vi "HFRR ADV v06.vi"() -> ()   [LabVIEW 2025] (continued)
            n2697 = Number To Fractional String(number=w3830, width (-)=i16 6, precision (6)=i16 2) -> (F-format string=w3835:string)  [unwired: 1 in]
            n2698 = Number To Fractional String(number=w3819, width (-)=i16 6, precision (6)=i16 2) -> (F-format string=w3821:string)  [unwired: 1 in]
            n2699 = Number To Fractional String(number=w3805, width (-)=i16 6, precision (6)=i16 2) -> (F-format string=w3806:string)  [unwired: 1 in]
            n2700 = Number To Fractional String(number=w3818, width (-)=i16 6, precision (6)=i16 2) -> (F-format string=w3820:string)  [unwired: 1 in]
            n2701 = Number To Fractional String(number=w3801, width (-)=i16 6, precision (6)=i16 2) -> (F-format string=w3800:string)  [unwired: 1 in]
            n2702 = Number To Fractional String(number=w3797, precision (6)=i16 2) -> (F-format string=w3796:string)  [unwired: 2 in]
            n2703 = call-dynamic "Set Report Header Text.vi"("report in"=w3839, "center header text"=w3791, "error in (no error)"=w3838) -> ("report out"=w3810:refnum<class "NI_report.lvclass">, "error out"=w3811:errorcluster)  [unwired: 11 in]
            n2704 = Concatenate Strings(w3799, w3783, w3835, w3799, w3780, w3804, w3799, w3778, w3817, w3799, w3775, w3806, w3799, w3771, w3821, w3799, w3768, w3820, w3799, w3766, w3800, w3799, w3763, w3796) -> (w3787:string)
            "export 2" <- w3787
            n2705 = call-poly <vilib>:"Append Report Text.vi"("report in"=w3810, "text"=w3809, "error in (no error)"=w3811) -> ("report out"=w3813:refnum<class "NI_report.lvclass">, "error out"=w3812:errorcluster)  [unwired: 9 in, 2 out]
            n2706 = local read "test by"() -> (w3786:string)
            n2707 = local read "TITTLE"() -> (w3788:string)
            n2708 = call-poly <vilib>:"Append Report Text.vi"("report in"=w3813, "error in (no error)"=w3812) -> ("report out"=w3834:refnum<class "NI_report.lvclass">, "error out"=w3832:errorcluster)  [unwired: 10 in, 2 out]
            n2709 = Concatenate Strings(w3788, w3787, w3786) -> (→"output":string)
            n2710 = call-poly <vilib>:"Append Report Text.vi"("report in"=w3834, "text"=w3787, "error in (no error)"=w3832) -> ("report out"=w3833:refnum<class "NI_report.lvclass">, "error out"=w3831:errorcluster)  [unwired: 9 in, 2 out]
            n2711 = call-dynamic "Print Report.vi"("report in"=w3833, "printer name (default)"=w3841, "error in (no error)"=w3831) -> ("report out"=w3843:refnum<class "NI_report.lvclass">, "error out"=w3844:errorcluster)  [unwired: 11 in]
            n2712 = call-dynamic "Dispose Report.vi"("report in"=w3843, "error in (no error)"=w3844) -> ()  [unwired: 13 in, 1 out]
          }
        }
        n2713 = case shown="True" "Print 2" {
          frame False {
          }
          frame True {
            n2714 = flat-sequence {
              frame #0 {
                n2715 = local read "s.NO"() -> (→"s.NO 2":string)
                n2716 = Wait (ms)(milliseconds to wait=u32 20) -> ()  [unwired: 1 out]
                n2717 = local read "Sample ID  3"() -> (→"Sample ID  6":string)
                n2718 = local read "Sample ID  4"() -> (→"Sample ID  7":string)
                n2719 = local read "Sample ID"() -> (→"Sample ID  2":string)
                n2720 = local read "Tested by"() -> (→"Tested by 2":string)
                n2721 = local read "Test Date"() -> (→"Test Date 2":string)
                n2722 = local read "Humidity after test 3"() -> (→"Humidity after test 4":dbl)
                n2723 = local read "Ref A Test Date :"() -> (→"TITTLE 4":string)
                n2724 = local read "Temperature before test 3"() -> (w3666:dbl)
                n2725 = local read "Temperature before test 3"() -> (→"Temperature after test 5":dbl)
                n2726 = local read "Temperature after test 3"() -> (→"Temperature after test 4":dbl)
                n2727 = local read "Humidity before test 3"() -> (→"Humidity before test 4":dbl)
                n2728 = local write "Temperature before test 3"(w3666) -> ()
                n2729 = local read "image data"() -> (w3657:T11)
                n2730 = String To Path(string="C:\\LAB-IQ\\im\\Temp_resized.jpg") -> (path=w3658:path)
                "path 2" <- w3658
                n2731 = call <vilib>:"Write JPEG File.vi"("image data"=w3657, "path to JPEG file"=w3658) -> ()  [unwired: 8 in, 2 out]
                "Ref A Test Date :" <- "Ref A Test Date :"
                "Ref B Test Date :" <- "Ref B Test Date :"
                "Ref B Scar Value :" <- "Ref B Scar Value :"
                "Ref A Scar Value :" <- "Ref A Scar Value :"
              }
              frame #1 {
                (unwired) HTML_Report_Image_Alignment."MIDDLE" ("alignment (default)")
                w3694 = u16 0 items=["portrait", "landscape"] ("orientation (portrait)")
                (unwired) HTML_Report_Image_Alignment."ABSMIDDLE" ("alignment (default)")
                (unwired) "TESTED BY : "
                (unwired) "TESTED DATE :"
                (unwired) "SAMPLE ID : "
                (unwired) "SAMPLE DESIGN : "
                w3727 = "\r"
                # "add image"
                n2732 = Wait (ms)(milliseconds to wait=u32 20) -> ()  [unwired: 1 out]
                n2733 = local read "Sample ID  2"() -> (w3720:string)
                n2734 = local read "Wear Scar X"() -> (w3692:dbl)
                "Length ( microns ) 2" <- w3692
                n2735 = local read "Wear Scar Y"() -> (w3691:dbl)
                "Wear Scar Y ( microns ) :" <- w3691
                n2736 = local read "Test Date 2"() -> (w3721:string)
                n2737 = local read "Tested by 2"() -> (w3722:string)
                n2738 = local read "String 46"() -> (w3718:string)
                n2739 = local read "String 48"() -> (w3724:string)
                n2740 = local read "String 47"() -> (w3723:string)
                n2741 = local read "String 49"() -> (w3725:string)
                n2742 = local read "String 10"() -> (w3678:string)
                n2743 = local read "s.NO 2"() -> (w3719:string)
                n2744 = Add(x=w3692, y=w3691) -> (x+y=w3690:dbl)
                n2745 = call <vilib>:"New Report.vi"("report type"=enum16{"Standard Report", "HTML"}."HTML") -> ("report out"=w3698:refnum<class "NI_report.lvclass">, "error out"=w3696:errorcluster)  [unwired: 13 in]
                n2746 = Concatenate Strings(w3727, w3718, w3719, w3727, w3724, w3720, w3727, w3723, w3721, w3727, w3725, w3722, w3727) -> (→"test by 2":string)
                n2747 = Concatenate Strings("C:\\LAB-IQ\\Data\\" ("string"), w3678, ".jpg" ("string")) -> ()  [unwired: 1 out]
                n2748 = Divide(x=w3690, y=2.0) -> (x/y=→"Mean Wear ( microns) :":dbl)
                n2749 = call-dynamic "Set Report Orientation.vi"("report in"=w3698, "orientation (portrait)"=w3694, "error in (no error)"=w3696) -> ("report out"=w3697:refnum<class "NI_report.lvclass">, "error out"=w3695:errorcluster)  [unwired: 11 in]
                n2750 = for {
                  N: 5 -> [_]
                  tunnel: w3697 -> [w3748]
                  tunnel: [w3747] -> w3676
                  tunnel: w3695 -> [w3746]
                  tunnel: [w3745] -> w3675
                  n2751 = call-dynamic "Set Report Tab Width.vi"("report in"=w3748, "error in (no error)"=w3746) -> ("report out"=w3747:refnum<class "NI_report.lvclass">, "error out"=w3745:errorcluster)  [unwired: 12 in]
                }
                n2752 = local read "TITTLE"() -> (w3693:string)
                n2753 = call-dynamic "Set Report Header Text.vi"("report in"=w3676, "center header text"=w3693, "error in (no error)"=w3675) -> ("report out"=w3714:refnum<class "NI_report.lvclass">, "error out"=w3713:errorcluster)  [unwired: 11 in]
                n2754 = for {
                  N: 1 -> [_]
                  tunnel: [w3752] -> w3700
                  tunnel: [w3751] -> w3699
                  tunnel: w3714 -> [w3750]
                  tunnel: w3713 -> [w3749]
                  n2755 = call-dynamic "New Report Line.vi"("report in"=w3750, "error in (no error)"=w3749) -> ("report out"=w3752:refnum<class "NI_report.lvclass">, "error out"=w3751:errorcluster)  [unwired: 12 in]
                }
                n2756 = for {
                  N: 2 -> [_]
                  tunnel: [w3744] -> w3706
                  tunnel: [w3743] -> w3705
                  tunnel: w3700 -> [w3742]
                  tunnel: w3699 -> [w3741]
                  n2757 = call-dynamic "New Report Line.vi"("report in"=w3742, "error in (no error)"=w3741) -> ("report out"=w3744:refnum<class "NI_report.lvclass">, "error out"=w3743:errorcluster)  [unwired: 12 in]
                }
                n2758 = for {
                  N: 25 -> [_]
                  tunnel: w3706 -> [w3740]
                  tunnel: w3705 -> [w3738]
                  tunnel: [w3739] -> w3709
                  tunnel: [w3737] -> w3708
                  n2759 = call-dynamic "Set Report Tab Width.vi"("report in"=w3740, "error in (no error)"=w3738) -> ("report out"=w3739:refnum<class "NI_report.lvclass">, "error out"=w3737:errorcluster)  [unwired: 12 in]
                }
                n2760 = control-ref of="Tab Control 9"() -> (w3704:refnum<vi>)
                n2761 = call-dynamic "Append Control Image to Report.vi"("report in"=w3709, "alignment (default)"=HTML_Report_Image_Alignment."ABSMIDDLE", "ctrl reference"=w3704, "error in (no error)"=w3708) -> ("report out"=w3703:refnum<class "NI_report.lvclass">, "error out"=w3702:errorcluster)  [unwired: 8 in, 2 out]
                n2762 = for {
                  N: 3 -> [_]
                  tunnel: [w3736] -> w3687
                  tunnel: [w3735] -> w3686
                  tunnel: w3703 -> [w3734]
                  tunnel: w3702 -> [w3733]
                  n2763 = call-dynamic "New Report Line.vi"("report in"=w3734, "error in (no error)"=w3733) -> ("report out"=w3736:refnum<class "NI_report.lvclass">, "error out"=w3735:errorcluster)  [unwired: 12 in]
                }
                n2764 = for {
                  N: 100 -> [_]
                  tunnel: w3687 -> [w3732]
                  tunnel: w3686 -> [w3730]
                  tunnel: [w3731] -> w3683
                  tunnel: [w3729] -> w3681
                  n2765 = call-dynamic "Set Report Tab Width.vi"("report in"=w3732, "error in (no error)"=w3730) -> ("report out"=w3731:refnum<class "NI_report.lvclass">, "error out"=w3729:errorcluster)  [unwired: 12 in]
                }
                n2766 = String To Path(string="C:\\LAB-IQ\\im\\Temp_resized.jpg") -> (path=w3673:path)
                n2767 = call-poly <vilib>:"Append Image to Report.vi"("report in"=w3683, "path or URL of image"=w3673, "error in (no error)"=w3681) -> ("report out"=w3682:refnum<class "NI_report.lvclass">, "error out"=w3680:errorcluster)  [unwired: 9 in, 2 out]
                n2768 = call-poly <vilib>:"Open HTML Report in Browser.vi"("report in"=w3682, "error in (no error)"=w3680) -> ("report out"=w3717:refnum<class "NI_report.lvclass">, "error out"=w3716:errorcluster)  [unwired: 11 in, 1 out]
                n2769 = call-dynamic "Dispose Report.vi"("report in"=w3717, "error in (no error)"=w3716) -> ()  [unwired: 13 in, 1 out]
              }
              frame #2 {
              }
              frame #3 {
                n2770 = disable-structure shown="Disabled" {
                  frame Disabled {
                    n2771 = local read "String 10"() -> (w3757:string)
                    n2772 = Concatenate Strings("C:\\LAB-IQ-NXT\\Data\\" ("string"), w3757, ".jpg" ("string")) -> (w3755:string)
                    n2773 = String To Path(string=w3755) -> (path=w3754:path)
                    n2774 = Delete(path (use dialog)=w3754) -> ()  [unwired: 4 in, 3 out]
                  }
                  frame Enabled {
                  }
                }
                n2775 = local write "Print 2"(FALSE ("Print")) -> ()
              }
            }
          }
        }
      }
    }
    n2776 = property on="SetTemp" class="DigNum (strict)"("Disabled"=w1732) -> ()  [unwired: 2 in, 2 out]
    n2777 = Multiply(x=w1721, y=w1723) -> (x*y=w1722:dbl)
    n2778 = local read "MWSD"() -> (w1720:dbl)
    n2779 = Add(x=w1722, y=w1720) -> (x+y=→"WS1.4":dbl)
    n2780 = Wait (ms)(milliseconds to wait=u32 50) -> ()  [unwired: 1 out]
    n2781 = Wait (ms)(milliseconds to wait=u32 50) -> ()  [unwired: 1 out]
    n2782 = local read "Quit"() -> (w1719:bool)
  }
  n2783 = VISA Close(VISA resource name=w44, error in (no error)=w43) -> (error out=w41:errorcluster)
  n2784 = VISA Close(VISA resource name=w25, error in (no error)=w24) -> ()  [unwired: 1 out]
  n2785 = call <vilib>:"Clear Errors.vi"("error in (no error)"=w41) -> ()  [unwired: 5 in, 2 out]
  n2786 = Or(x=w31, y=w30) -> (x .or. y?=w32:bool)
  n2787 = while {
    tunnel: [w3905] -> w37
    shift-right: [w3943] -> _
    shift-left: "" -> [w3931]
    tunnel: [w3919] -> _
    i -> [w3919]
    stop <- w3905 stop-if-true
    w3945 = ";" ("string")
    n2788 = local read "start en"() -> (w3964:bool)
    n2789 = And(x="st enable", y=w3964) -> (x .and. y?=w3965:bool)
    n2790 = local read "ACQUIRE 3"() -> (w3908:bool)
    n2791 = local read "Elapsed time"() -> (w3927:dbl)
    n2792 = case shown="True" w3965 {
      tunnel: "st enable" -> [w4029 w4030]
      tunnel: [w4029 w4030] -> w3909
      frame False {
      }
      frame True {
        n2793 = local write "start en"(FALSE ("start en")) -> ()
      }
    }
    n2794 = Wait (ms)(milliseconds to wait=u32 80) -> ()  [unwired: 1 out]
    n2795 = local read "Stroke"() -> (w3918:dbl)
    n2796 = Greater?(x=w3927, y=0.1) -> (0:w3925:bool)
    n2797 = Or(x=w3909, y=w3908) -> (x .or. y?=w3910:bool)
    n2798 = case shown="True" "ACQUIRE 2" {
      frame False {
      }
      frame True {
        n2799 = call "Elapsed Time13"() -> ("Time has Elapsed"=w3972:bool)  [unwired: 12 in, 7 out]
        n2800 = case shown="True" w3972 {
          frame False {
          }
          frame True {
            n2801 = local write "ACQUIRE 2"(FALSE ("ACQUIRE 2")) -> ()
            n2802 = local write "ACQUIRE 3"(FALSE ("ACQUIRE 2")) -> ()
          }
        }
        n2803 = local write "ACQUIRE 3"(TRUE ("ACQUIRE 2")) -> ()
      }
    }
    n2804 = case shown="True" w3910 {
      tunnel: w3918 -> [_ w4052]
      tunnel: [w4032 _] -> w3962
      tunnel: w3925 -> [_ _]
      tunnel: w3908 -> [_ w4039]
      frame False {
        w4032 = TRUE ("PID Rst")
        n2805 = local read "stop cmd"() -> (w4033:bool)
        n2806 = case shown="True" w4033 {
          frame False {
          }
          frame True {
            n2807 = local write "stop cmd"(FALSE ("stop cmd")) -> ()
          }
        }
        n2808 = local write "PID Rst"(TRUE ("PID Rst")) -> ()
        "start en" <- w4032
      }
      frame True {
        w4059 = cluster{"output high":dbl, "output low":dbl} {"output high"=600.0, "output low"=-600.0} ("output range")
        n2809 = local read "STROKE GAIN :"() -> (w4044:dbl)
        n2810 = call "Elapsed Time6"("Reset"="PID Rst", "Auto Reset"=FALSE) -> ("Time has Elapsed"=w4053:bool)  [unwired: 10 in, 7 out]
        n2811 = Multiply(x="Set Strk", y=w4044) -> (x*y=w4037:dbl)
        n2812 = case shown="False" w4053 {
          tunnel: [w4064 w4065] -> w4056
          tunnel: "Set Strk" -> [w4064 _]
          tunnel: w4052 -> [_ w4065]
          frame False {
          }
          frame True {
          }
        }
        n2813 = Multiply(x=w4037, y=1.0) -> (x*y=w4036:dbl)
        n2814 = Select(t=T8 {"Proportional Gain (Kc)"=0.0, "Integral Time (Ti, min)"=0.02, "Derivative Time (Td, min)"=0.0} ("Stroke PID Gains"), s=w4039, f="Stroke PID Gains") -> (s? t:f=w4040:T8)
        n2815 = Not(x=w4053) -> (.not. x?=w4051:bool)
        n2816 = call-poly <vilib>:"PID.vi"("reinitialize? (F)"=w4051, "output range"=w4059, "PID gains"=w4040, "process variable"=w4056, "setpoint"="Set Strk") -> ("output"=w4050:dbl)  [unwired: 5 in, 1 out]
        "Slide 5" <- w4050
        n2817 = Select(t=w4050, s=w4053, f=0.0) -> (s? t:f=w4054:dbl)
        n2818 = flat-sequence {
          tunnel: w4054 -> [_]
          frame #0 {
            n2819 = local write "PID Rst"(FALSE ("PID Rst")) -> ()
          }
        }
        n2820 = Add(x=w4036, y=w4054) -> (x+y=w4049:dbl)
        n2821 = Unbundle(w4059) -> ("output high"=w4058:dbl, "output low"=w4057:dbl)
        n2822 = To Word Integer(number=w4049) -> (16bit integer=w4046:i16)
        n2823 = property on="Slide 5" class="Slide (strict)"("Scale.Range:Minimum"=w4057, "Scale.Range:Maximum"=w4058) -> ()  [unwired: 2 in, 2 out]
        n2824 = In Range and Coerce(upper limit=4095.0 ("f"), x=w4046, lower limit=100.0 ("f")) -> (coerced(x)=w4043:dbl)  [unwired: 1 out]
        "PID Out" <- w4043
        n2825 = Number To Decimal String(number=w4043) -> (decimal integer string=→"st gain":string)  [unwired: 1 in]
        "stop cmd" <- TRUE ("Auto Reset")
      }
    }
    n2826 = flat-sequence {
      frame #0 {
        n2827 = local read "CH-POWER +"() -> (w3976:u16)
        n2828 = local read "CH-POWER -"() -> (w3977:u16)
        n2829 = case shown="1" w3977 {
          tunnel: "PWR" -> [w3978 w3979 w3980 w3981 w3982 w3983 w3984 w3985]
          frame 0, Default {
            n2830 = local write "Do 0"(w3978) -> ()
          }
          frame 1 {
            n2831 = local write "Do 1"(w3979) -> ()
          }
          frame 2 {
            n2832 = local write "Do 2"(w3980) -> ()
          }
          frame 3 {
            n2833 = local write "Do 3"(w3981) -> ()
          }
          frame 4 {
            n2834 = local write "Do 4"(w3982) -> ()
          }
          frame 5 {
            n2835 = local write "Do 5"(w3983) -> ()
          }
          frame 6 {
            n2836 = local write "Do 6"(w3984) -> ()
          }
          frame 7 {
            n2837 = local write "Do 7"(w3985) -> ()
          }
        }
        n2838 = case shown="1" w3976 {
          tunnel: "PWR" -> [w3986 w3987 w3988 w3989 w3990 w3991 w3992 w3993]
          frame 0, Default {
            n2839 = local write "Do 0"(w3986) -> ()
          }
          frame 1 {
            n2840 = local write "Do 1"(w3987) -> ()
          }
          frame 2 {
            n2841 = local write "Do 2"(w3988) -> ()
          }
          frame 3 {
            n2842 = local write "Do 3"(w3989) -> ()
          }
          frame 4 {
            n2843 = local write "Do 4"(w3990) -> ()
          }
          frame 5 {
            n2844 = local write "Do 5"(w3991) -> ()
          }
          frame 6 {
            n2845 = local write "Do 6"(w3992) -> ()
          }
          frame 7 {
            n2846 = local write "Do 7"(w3993) -> ()
          }
        }
      }
    }
    n2847 = local read "RUN"() -> (w3916:bool)
    n2848 = Or(x=w3916, y="ACQUIRE 3") -> (x .or. y?=w3915:bool)
    n2849 = local read "Set Hz"() -> (w3933:dbl)
    n2850 = Select(t=w3933, s=w3915, f=0.0) -> (s? t:f=w3932:dbl)
    n2851 = local read "st gain"() -> (w3936:string)
    n2852 = local read "DO"() -> (w3937:string)
    n2853 = case shown="True" "Boolean 10" {
      frame False {
      }
      frame True {
        n2854 = local write "Tab Control 8"(enum32{"setup", "calibrate"}."calibrate" ("Tab Control 8")) -> ()
        n2855 = local write "Boolean 10"(FALSE ("Boolean 10")) -> ()
      }
    }
    n2856 = Number To Decimal String(number=w3932) -> (decimal integer string=w3935:string)  [unwired: 1 in]
    n2857 = case shown="True" "Boolean 11" {
      frame False {
      }
      frame True {
        n2858 = local write "Tab Control 8"(enum32{"setup", "calibrate"}."setup" ("Tab Control 8")) -> ()
        n2859 = local write "Boolean 11"(FALSE ("Boolean 11")) -> ()
      }
    }
    n2860 = String Length(string=w3936) -> (length=w3951:i32)
    n2861 = String Length(string=w3937) -> (length=w3939:i32)
    n2862 = String Length(string=w3935) -> (length=w3952:i32)
    n2863 = Subtract(x=4.0, y=w3951) -> (x-y=w3948:dbl)
    n2864 = Subtract(x=3.0, y=w3939) -> (x-y=w3942:dbl)
    n2865 = flat-sequence {
      tunnel: w3962 -> [_]
      frame #0 {
        n2866 = Build Array("Do 0", "Do 1", "Do 2", "Do 3", "Do 4", "Do 5", "Do 6", "Do 7") -> (w4020:bool[])
        n2867 = Boolean Array To Number(Boolean array=w4020) -> (number=w4018:u32)
        n2868 = Add(x=w4018, y=u32 0) -> (x+y=w4016:u32)
        n2869 = Number To Decimal String(number=w4016) -> (decimal integer string=→"DO":string)  [unwired: 1 in]
      }
    }
    n2870 = Subtract(x=3.0, y=w3952) -> (x-y=w3953:dbl)
    n2871 = Replace Substring(3:w3948, 4:w3936, 5:"0000" ("string")) -> (1:w3946:string)  [unwired: 1 in, 1 out]
    n2872 = Replace Substring(3:w3942, 4:w3937, 5:"000" ("string")) -> (1:w3938:string)  [unwired: 1 in, 1 out]
    n2873 = Replace Substring(3:w3953, 4:w3935, 5:"000" ("string")) -> (1:w3947:string)  [unwired: 1 in, 1 out]
    n2874 = Concatenate Strings("*" ("string"), w3947, w3945, w3946, w3945, w3938, "$" ("string")) -> (w3943:string)
    "Stroke_send_Val" <- w3943
    n2875 = local read "RUN"() -> (w3913:bool)
    n2876 = local read "ACQUIRE 3"() -> (w3912:bool)
    n2877 = local read "send"() -> (w3929:bool)
    n2878 = Not Equal?(x=w3931, y=w3943) -> (x != y?=w3944:bool)
    n2879 = Or(x=w3913, y=w3912) -> (x .or. y?=w3911:bool)
    n2880 = And(x=w3929, y=w3911) -> (x .and. y?=w3928:bool)
    n2881 = Or(x=w3944, y=w3928) -> (x .or. y?=w3922:bool)
    n2882 = case shown="False" w3911 {
      frame False {
        "send" <- TRUE ("send")
      }
      frame True {
      }
    }
    n2883 = call "Elapsed Time4"("Time Target (s)"=0.5) -> ("Time has Elapsed"=w3920:bool)  [unwired: 11 in, 7 out]
    n2884 = local read "Din"() -> (w3961:u8[])
    n2885 = Or(x=w3920, y=w3922) -> (x .or. y?=w3921:bool)
    n2886 = local read "Quit"() -> (w3905:bool)
    n2887 = Index Array(array=w3961, index=0) -> (element=w3959:u8)
    n2888 = case shown="True" w3921 {
      tunnel: w3943 -> [_ w3997]
      frame False {
      }
      frame True {
        n2889 = local read "Due Com"() -> (w3998:string[])
        n2890 = Build Array (concatenate)(w3998, w3997) -> (→"Due Com":string[])
        n2891 = local write "send"(FALSE ("send")) -> ()
      }
    }
    n2892 = Number To Boolean Array(number=w3959) -> (Boolean array=w3958:bool[])
    n2893 = Array Size(array=w3958) -> (size(s)=w3957:i32)
    n2894 = Greater Than 0?(x=w3957) -> (x > 0?=w3956:bool)
    n2895 = case shown="True" w3956 {
      tunnel: w3958 -> [_ w4012]
      frame False {
      }
      frame True {
        n2896 = Index Array(array=w4012, index #1=0 ("index"), index #2=1 ("index"), index #3=2 ("index"), index #4=3 ("index"), index #5=4 ("index"), index #6=5 ("index"), index #7=6 ("index"), index #8=7 ("index")) -> (element #1=→"DI 0":bool, element #2=→"DI 1":bool, element #3=→"DI 2":bool, element #4=→"DI 3":bool, element #5=→"DI 4":bool, element #6=→"DI 5":bool, element #7=→"DI 6":bool, element #8=→"DI 7":bool)
      }
    }
  }
  n2897 = Or(x=w27, y=w32) -> (x .or. y?=w39:bool)
  n2898 = control-ref of="new picture"() -> ()  [unwired: 1 out]
  n2899 = Or(x=w46, y=w39) -> (x .or. y?=w36:bool)
  n2900 = Or(x=w36, y=w37) -> (x .or. y?=w28:bool)
  n2901 = while {
    tunnel: [w4067] -> w50
    tunnel: [w4068] -> _
    i -> [w4068]
    stop <- w4067 stop-if-true
    n2902 = local read "PID-out"() -> (w4069:dbl)
    "Horizontal Slider Control" <- w4069
    n2903 = Greater Or Equal?(x=w4069, y=2.0) -> (x >= y?=w4070:bool)
    n2904 = flat-sequence {
      tunnel: w4070 -> [w4078]
      tunnel: w4069 -> [w4081]
      tunnel: [w4079] -> w4076
      tunnel: [w4077] -> w4075
      tunnel: [w4097] -> w4074
      tunnel: w4076 -> [w4097]
      tunnel: w4075 -> [w4094]
      tunnel: [w4094] -> w4073
      tunnel: w4074 -> [w4099]
      tunnel: [w4098] -> w4072
      tunnel: w4073 -> [w4098]
      tunnel: w4072 -> [w4113]
      frame #0 {
        n2905 = case shown="True" w4078 {
          selector: w4078 -> [w4083 _]
          frame False {
            n2906 = local write "HEATER"(w4083) -> ()
          }
          frame True {
            w4085 = TRUE ("data")
            n2907 = local read "CH-HEATER"() -> (w4084:u16)
            n2908 = case shown="2" w4084 {
              tunnel: w4085 -> [w4086 w4087 w4088 w4089 w4090 w4091 w4092 w4093]
              frame 0, Default {
                n2909 = local write "Do 0"(w4086) -> ()
              }
              frame 1 {
                n2910 = local write "Do 1"(w4087) -> ()
              }
              frame 2 {
                n2911 = local write "Do 2"(w4088) -> ()
              }
              frame 3 {
                n2912 = local write "Do 3"(w4089) -> ()
              }
              frame 4 {
                n2913 = local write "Do 4"(w4090) -> ()
              }
              frame 5 {
                n2914 = local write "Do 5"(w4091) -> ()
              }
              frame 6 {
                n2915 = local write "Do 6"(w4092) -> ()
              }
              frame 7 {
                n2916 = local write "Do 7"(w4093) -> ()
              }
            }
            "HEATER" <- w4085
          }
        }
        n2917 = Select(t=w4081, s=w4078, f=0.0) -> (s? t:f=w4077:dbl)
        n2918 = Greater Or Equal?(x=w4081, y=97.0) -> (x >= y?=w4079:bool)
      }
      frame #1 {
        n2919 = Multiply(x=w4094, y=5.0) -> (x*y=w4096:dbl)
        n2920 = Wait (ms)(milliseconds to wait=w4096) -> ()  [unwired: 1 out]
      }
      frame #2 {
        n2921 = case shown="False" w4099 {
          frame False {
            w4100 = FALSE ("data")
            n2922 = local read "CH-HEATER"() -> (w4101:u16)
            n2923 = case shown="4" w4101 {
              tunnel: w4100 -> [w4102 w4103 w4104 w4105 w4106 w4107 w4108 w4109]
              frame 0, Default {
                n2924 = local write "Do 0"(w4102) -> ()
              }
              frame 1 {
                n2925 = local write "Do 1"(w4103) -> ()
              }
              frame 2 {
                n2926 = local write "Do 2"(w4104) -> ()
              }
              frame 3 {
                n2927 = local write "Do 3"(w4105) -> ()
              }
              frame 4 {
                n2928 = local write "Do 4"(w4106) -> ()
              }
              frame 5 {
                n2929 = local write "Do 5"(w4107) -> ()
              }
              frame 6 {
                n2930 = local write "Do 6"(w4108) -> ()
              }
              frame 7 {
                n2931 = local write "Do 7"(w4109) -> ()
              }
            }
            n2932 = local write "HEATER"(w4100) -> ()
          }
          frame True {
          }
        }
      }
      frame #3 {
        n2933 = Subtract(x=100, y=w4113) -> (x-y=w4112:dbl)
        n2934 = Multiply(x=w4112, y=5.0) -> (x*y=w4110:dbl)
        n2935 = Wait (ms)(milliseconds to wait=w4110) -> ()  [unwired: 1 out]
      }
    }
    n2936 = local read "Quit"() -> (w4067:bool)
  }
  n2937 = Or(x=w50, y=w28) -> (x .or. y?=w49:bool)
  n2938 = while {
    tunnel: [w4115] -> w45
    i -> [w4122]
    stop <- w4115 stop-if-true
    n2939 = local read "Quit"() -> (w4115:bool)
    n2940 = Equal To 0?(x=w4122) -> (x = 0?=w4120:bool)
    n2941 = call "Elapsed Time3"("Time Target (s)"=45.0, "Auto Reset"=TRUE) -> ("Time has Elapsed"=w4119:bool)  [unwired: 10 in, 7 out]
    n2942 = Wait (ms)(milliseconds to wait=u32 50) -> ()  [unwired: 1 out]
    n2943 = Or(x=w4119, y=w4120) -> (x .or. y?=w4121:bool)
    n2944 = case shown="True" w4121 {
      frame False {
      }
      frame True {
        n2945 = call <vilib>:"System Exec.vi"("run minimized? (F)"=TRUE, "error in (no error)"="error in (no error)", "command line"="powercfg.exe -change -monitor-timeout-ac 0") -> ("error out"=w4133:errorcluster)  [unwired: 5 in, 3 out]
        n2946 = call <vilib>:"System Exec.vi"("run minimized? (F)"=TRUE, "error in (no error)"=w4133, "command line"="powercfg.exe -change -disk-timeout-ac 0") -> ("error out"=w4132:errorcluster)  [unwired: 5 in, 3 out]
        n2947 = call <vilib>:"System Exec.vi"("run minimized? (F)"=TRUE, "error in (no error)"=w4132, "command line"="powercfg.exe -change -standby-timeout-ac 0") -> ("error out"=w4131:errorcluster)  [unwired: 5 in, 3 out]
        n2948 = call <vilib>:"System Exec.vi"("run minimized? (F)"=TRUE, "error in (no error)"=w4131, "command line"="powercfg.exe -change -hibernate-timeout-ac 0") -> ("error out"=w4130:errorcluster)  [unwired: 5 in, 3 out]
        n2949 = call <vilib>:"Simple Error Handler.vi"("error in (no error)"=w4130) -> ("error out"=w4136:errorcluster)  [unwired: 4 in, 4 out]
        n2950 = call <vilib>:"Clear Errors.vi"("error in (no error)"=w4136) -> ("error out"=→"error out":errorcluster)  [unwired: 5 in, 1 out]
      }
    }
  }
  n2951 = Compound Arithmetic op=OR(w48, w49, w45) -> (w47:bool)
  n2952 = flat-sequence {
    tunnel: w47 -> [_]
    tunnel: [w4138] -> w3
    tunnel: w3 -> [_]
    frame #0 {
      n2953 = call "CLOSE CONNECTION.vi"() -> ("error out"=w4138:errorcluster)  [unwired: 11 in]
    }
    frame #1 {
      n2954 = Quit LabVIEW(quit? (T)=TRUE) -> ()
      n2955 = local write "Quit"(FALSE ("EXIT")) -> ()
    }
  }
  n2956 = property on="Heater Button" class="Bool (strict)"("Visible"=TRUE) -> ()  [unwired: 2 in, 2 out]
  n2957 = disable-structure shown="Disabled" {
    disable-tunnel: _ -> [w4144 _]
    disable-tunnel: _ -> [w4141 _]
    disable-tunnel: _ -> [w4142 _]
    frame Disabled {
      n2958 = disable-structure shown="Disabled" {
        disable-tunnel: [w4151 _] -> w4143
        frame Disabled {
          n2959 = while {
            shift-right: [w4193] -> w4149
            shift-left: errorcluster {"status"=TRUE, "code"=0, "source"="Init"} ("error out") -> [w4158]
            shift-right: [w4192] -> w4148
            shift-left: _ -> [w4159]
            shift-right: [w4191] -> _
            shift-left: "" -> [w4190]
            tunnel: [w4152] -> w4151
            shift-right: ["Set Rh"] -> _
            shift-left: 0.0 ("Set Rh") -> [w4184]
            tunnel: [w4161] -> _
            i -> [w4161]
            stop <- w4152 stop-if-true
            n2960 = flat-sequence {
              tunnel: w4158 -> [w4196]
              tunnel: [w4196] -> w4157
              frame #0 {
                n2961 = Wait (ms)(milliseconds to wait=u32 200) -> ()  [unwired: 1 out]
              }
            }
            n2962 = local read "Com Port 3"() -> (w4160:refnum<visa-resource-name>)
            n2963 = local read "Humidity Str Rec"() -> (w4162:string)
            n2964 = Not Equal?(x="Set Rh", y=w4184) -> (x != y?=w4189:bool)
            n2965 = Number To Decimal String(number="Set Rh") -> (decimal integer string=w4187:string)  [unwired: 1 in]
            n2966 = Not Equal?(x=w4160, y=w4159) -> (x != y?=w4155:bool)
            n2967 = Concatenate Strings("#setPoint00" ("string"), w4187) -> (w4188:string)
            n2968 = case shown="False" w4189 {
              tunnel: w4188 -> [_ w4208]
              frame False {
                n2969 = local read "Humidity"() -> (w4205:bool)
                n2970 = case shown="True" w4205 {
                  frame False {
                    n2971 = local write "Humidity Str Send"("stop" ("Humidity Str Send")) -> ()
                  }
                  frame True {
                    n2972 = local write "Humidity Str Send"("start" ("Humidity Str Send")) -> ()
                  }
                }
              }
              frame True {
                n2973 = local write "Humidity Str Send"(w4208) -> ()
              }
            }
            n2974 = Or(x=w4155, y="Re-Initialise") -> (x .or. y?=w4154:bool)
            n2975 = String Subset(string=w4162, offset (0)=7) -> (substring=w4177:string)  [unwired: 1 in]
            n2976 = Match Pattern(string=w4162, regular expression="?") -> (offset past match=w4180:i32)  [unwired: 1 in, 3 out]
            n2977 = Match Pattern(string=w4162, regular expression="v") -> (offset past match=w4183:i32)  [unwired: 1 in, 3 out]
            n2978 = case shown="True" w4154 {
              tunnel: w4157 -> [w4194 _]
              tunnel: [w4194 errorcluster {"status"=TRUE, "code"=0, "source"="Init"} ("error out")] -> w4156
              frame False {
              }
              frame True {
              }
            }
            n2979 = Equal?(x=w4180, y=-1) -> (x = y?=w4164:bool)
            n2980 = Match Pattern(string=w4177, regular expression="g") -> (after substring=w4178:string, offset past match=w4169:i32)  [unwired: 1 in, 2 out]
            n2981 = Match Pattern(string=w4177, regular expression="y") -> (after substring=w4176:string, offset past match=w4170:i32)  [unwired: 1 in, 2 out]
            n2982 = Greater?(x=w4170, y=w4169) -> (0:w4175:bool)
            n2983 = Greater Or Equal To 0?(x=w4170) -> (x >= 0?=w4167:bool)
            n2984 = Greater Or Equal To 0?(x=w4169) -> (x >= 0?=w4168:bool)
            n2985 = Or(x=w4167, y=w4168) -> (x .or. y?=w4166:bool)
            n2986 = Greater Or Equal To 0?(x=w4183) -> (x >= 0?=w4165:bool)
            n2987 = Select(t=w4176, s=w4175, f=w4178) -> (s? t:f=w4171:string)
            n2988 = case shown="Error" w4156 {
              selector: w4156 -> [w4221 w4267]
              tunnel: [w4219 w4260] -> w4193
              tunnel: w4159 -> [w4222 w4266]
              tunnel: [w4220 w4269] -> w4192
              tunnel: w4190 -> [w4209 w4268]
              tunnel: [w4216 w4268] -> w4191
              frame No Error {
                n2989 = call "Elapsed Time7"() -> ("Time has Elapsed"=w4215:bool)  [unwired: 12 in, 7 out]
                n2990 = Not Equal?(x="Humidity Str Send", y=w4209) -> (x != y?=w4211:bool)
                n2991 = Or(x=w4211, y=w4215) -> (x .or. y?=w4214:bool)
                n2992 = Select(t="Humidity Str Send", s=w4211, f="vals" ("regular expression")) -> (s? t:f=w4210:string)
                n2993 = Or(x=w4214, y="Send") -> (x .or. y?=w4218:bool)
                n2994 = case shown="True" w4218 {
                  tunnel: [w4225 w4230] -> w4219
                  tunnel: w4222 -> [w4224 w4238]
                  tunnel: w4221 -> [w4225 w4237]
                  tunnel: [w4224 w4231] -> w4220
                  tunnel: w4210 -> [_ w4236]
                  tunnel: [w4223 w4227] -> w4216
                  tunnel: "Humidity Str Send" -> [_ w4228]
                  tunnel: w4211 -> [_ w4229]
                  tunnel: w4209 -> [w4223 w4226]
                  frame False {
                  }
                  frame True {
                    n2995 = flat-sequence {
                      tunnel: w4238 -> [w4246]
                      tunnel: w4237 -> [w4245]
                      tunnel: w4236 -> [w4242]
                      tunnel: [w4244] -> w4235
                      tunnel: [w4243] -> w4234
                      tunnel: w4235 -> [w4249]
                      tunnel: w4234 -> [w4248]
                      tunnel: [w4249] -> w4233
                      tunnel: [w4248] -> w4232
                      tunnel: w4233 -> [w4256]
                      tunnel: w4232 -> [w4255]
                      tunnel: [w4254] -> w4231
                      tunnel: [w4253] -> w4230
                      frame #0 {
                        n2996 = local write "Ser Led"(TRUE ("Boolean 4")) -> ()
                        n2997 = Concatenate Strings(w4242, "\r") -> (w4241:string)
                        n2998 = VISA Write(VISA resource name=w4246, write buffer=w4241, error in (no error)=w4245) -> (VISA resource name out=w4244:refnum<visa-resource-name>, error out=w4243:errorcluster)  [unwired: 1 out]
                      }
                      frame #1 {
                        n2999 = Wait (ms)(milliseconds to wait="wait") -> ()  [unwired: 1 out]
                      }
                      frame #2 {
                        w4251 = FALSE ("Send")
                        n3000 = property class="Instr"(reference=w4256, error in=w4255) -> (reference out=w4257:refnum<visa-resource-name>, error out=w4258:errorcluster, "Serial Settings:Number of Bytes at Serial Port"=w4250:u32)
                        "Humidity 2" <- w4250
                        n3001 = local write "Send"(w4251) -> ()
                        n3002 = local write "Ser Led"(w4251) -> ()
                        n3003 = VISA Read(VISA resource name=w4257, byte count=w4250, error in (no error)=w4258) -> (VISA resource name out=w4254:refnum<visa-resource-name>, read buffer=→"Humidity Str Rec":string, error out=w4253:errorcluster)  [unwired: 1 out]
                      }
                    }
                    n3004 = Select(t=w4228, s=w4229, f=w4226) -> (s? t:f=w4227:string)
                  }
                }
              }
              frame Error {
                w4274 = u16 0 items=["None"=0, "XON/XOFF"=1, "RTS/CTS"=2, "DTR/DSR"=4] ("flow control")
                w4270 = u16 0 items=["None", "Odd", "Even", "Mark", "Space"] ("parity")
                w4273 = u16 10 items=["1.0"=10, "1.5"=15, "2.0"=20] ("stop bits")
                n3005 = VISA Close(VISA resource name=w4266, error in (no error)=w4267) -> (error out=w4265:errorcluster)
                n3006 = local write "humid"("" ("humid")) -> ()
                n3007 = local write "Humidity Str Rec"("" ("Humidity Str Rec")) -> ()
                n3008 = call <vilib>:"Clear Errors.vi"("error in (no error)"=w4265) -> ("error out"=w4264:errorcluster)  [unwired: 5 in, 1 out]
                n3009 = local read "Com Port 3"() -> (w4263:refnum<visa-resource-name>)
                n3010 = call-poly "VISA Configure Serial Port"("VISA resource name"=w4263, "timeout (10sec)"=u32 1000, "termination char\n(0xA = '\\n' = LF)"=u8 10 ("termination char\n(0xA = '\\n' = LF)"), "Enable Termination\nChar (T)"=FALSE ("Enable Termination Char (T)"), "baud rate (9600)"="Humidity BaudRate", "data bits (8)"=u16 8 ("data bits"), "parity (0:none)"=w4270, "error in (no error)"=w4264, "stop bits (10: 1 bit)"=w4273, "flow control (0:none)"=w4274) -> ("VISA resource name out"=w4269:refnum<visa-resource-name>, "error out"=w4260:errorcluster)  [unwired: 4 in]
              }
            }
            n3011 = Compound Arithmetic op=AND(w4165, w4164, w4166) -> (w4163:bool)
            n3012 = case shown="True" w4163 {
              tunnel: w4162 -> [_ _]
              tunnel: w4171 -> [_ w4201]
              frame False {
              }
              frame True {
                w4199 = " " ("regular expression")
                n3013 = Match Pattern(string=w4201, regular expression=" ") -> (after substring=w4203:string)  [unwired: 1 in, 3 out]
                n3014 = Match Pattern(string=w4203, regular expression=w4199) -> (before substring=→"humid":string, after substring=w4200:string)  [unwired: 1 in, 2 out]
                n3015 = Match Pattern(string=w4200, regular expression=w4199) -> (before substring=→"temp_@Rh sensor":string)  [unwired: 1 in, 3 out]
              }
            }
            n3016 = local read "Quit"() -> (w4152:bool)
          }
          n3017 = VISA Close(VISA resource name=w4148, error in (no error)=w4149) -> (error out=w4145:errorcluster)
          n3018 = call <vilib>:"Clear Errors.vi"("error in (no error)"=w4145) -> ()  [unwired: 5 in, 2 out]
        }
        frame Enabled {
        }
      }
    }
    frame Enabled {
    }
  }
  n3019 = while {
    tunnel: [w4282] -> _
    i -> [w4282]
    stop <- w4277 stop-if-true
    # "Langauage selection"
    n3020 = property on="FF Calibration g" class="WFGraph (strict)"("Plot Area:Colors:FG Color"=u32 0) -> ()  [unwired: 2 in, 2 out]
    n3021 = Equal?(x="Lan flag", y=22.0) -> ()  [unwired: 1 out]
    n3022 = disable-structure shown="Disabled" {
      frame Disabled {
        n3023 = stacked-sequence {
          frame #0 {
            n3024 = case shown="\"Russian\"" "Language Selection" {
              tunnel: [0 1] -> w4284
              frame "English", Default {
              }
              frame "Russian" {
              }
            }
            n3025 = for {
              N: 130 -> [_]
              tunnel: "Table" -> [w4293]
              tunnel: w4284 -> [w4292]
              i -> [w4291]
              n3026 = Index Array(array=w4293, index (row)=w4291, index (col)=w4292) -> (element=w4290:string)
              n3027 = case shown="123" w4291 {
                tunnel: w4290 -> [w4294 w4295 _ w4296 w4297 w4298 w4299 w4300 w4301 w4302 w4303 w4304 w4305 w4306 w4307 w4308 w4309 w4310 w4311 w4312 w4313 w4314 w4315 w4316 w4317 w4318 w4319 w4320 w4321 _ _ w4322 w4323 w4324 w4325 w4326 w4327 w4336 w4343 w4350 w4357 w4361 w4364 w4367 w4369 w4371 w4372 w4373 w4374 w4375 w4376 w4377 w4378 w4379 w4380 w4381 w4382 w4383 w4384 w4385 w4386 w4387 w4388 w4389 w4390 w4391 w4392 w4393 w4394 w4395 w4396 w4397 w4398 w4399 w4400 w4401 w4402 w4403 w4404 w4405 w4406 w4407 w4408 w4409 w4410 w4411 w4412 w4413 w4414 w4415 w4416 w4417 w4418 w4419 w4420 w4421 w4422 w4423 w4424 w4425 w4426 w4427 w4428 w4429 w4430 _ w4431 w4432 w4433 w4434 w4435 w4436 w4437 w4438 w4439 w4440 w4441 w4442 w4443 _ w4444 w4445 w4446 w4447 w4448 w4449 _]
                frame 0 {
                  n3028 = local write "S"(w4294) -> ()
                }
                frame 1 {
                  n3029 = local write "S 2"(w4295) -> ()
                }
                frame 2 {
                }
                frame 3 {
                  n3030 = local write "S 4"(w4296) -> ()
                }
                frame 4 {
                  n3031 = property on="FILE" class="Str"("Caption.Text"=w4297) -> ()  [unwired: 2 in, 2 out]
                }
                frame 5 {
                  n3032 = property on="Fuel Discription :" class="Str"("Caption.Text"=w4298) -> ()  [unwired: 2 in, 2 out]
                }
                frame 6 {
                  n3033 = property on="Remarks :" class="Str"("Caption.Text"=w4299) -> ()  [unwired: 2 in, 2 out]
                }
                frame 7 {
                  n3034 = property on="Save & Continue" class="Bool (strict)"("Boolean Text.Text"=w4300) -> ()  [unwired: 2 in, 2 out]
                }
                frame 8 {
                }
                frame 9 {
                  n3035 = property on="Set Hz" class="DigNum (strict)"("Caption.Text"=w4302) -> ()  [unwired: 2 in, 2 out]
                }
                frame 10 {
                  "String 3" <- w4303
                }
                frame 11 {
                  n3036 = property on="NORMAL LOAD" class="DigNum (strict)"("Caption.Text"=w4304) -> ()  [unwired: 2 in, 2 out]
                }
                frame 12 {
                  "String 5" <- w4305
                }
                frame 13 {
                  n3037 = property on="Set Temp" class="DigNum (strict)"("Caption.Text"=w4306) -> ()  [unwired: 2 in, 2 out]
                }
                frame 14 {
                  n3038 = local write "S 15"(w4307) -> ()
                }
                frame 15 {
                  n3039 = property on="Set Rh" class="DigNum (strict)"("Caption.Text"=w4308) -> ()  [unwired: 2 in, 2 out]
                }
                frame 16 {
                  "String 13" <- w4309
                  "String 26" <- w4309
                }
                frame 17 {
                  n3040 = local write "S 18"(w4310) -> ()
                }
                frame 18 {
                  "String 17" <- w4311
                }
                frame 19 {
                  n3041 = property on="test time" class="DigNum (strict)"("Caption.Text"=w4312) -> ()  [unwired: 2 in, 2 out]
                }
                frame 20 {
                  "String 18" <- w4313
                  "String 22" <- w4313
                }
                frame 21 {
                  n3042 = property on="Elapsed time" class="DigNum (strict)"("Caption.Text"=w4314) -> ()  [unwired: 2 in, 2 out]
                }
                frame 22 {
                  n3043 = property on="Samplingtime 2" class="DigNum (strict)"("Caption.Text"=w4315) -> ()  [unwired: 2 in, 2 out]
                }
                frame 23 {
                  "String 21" <- w4316
                }
                frame 24 {
                  n3044 = property on="Countdown" class="DigNum (strict)"("Caption.Text"=w4317) -> ()  [unwired: 2 in, 2 out]
                }
                frame 25 {
                  n3045 = property on="Countdown 2" class="DigNum (strict)"("Caption.Text"=w4318) -> ()  [unwired: 2 in, 2 out]
                }
                frame 26 {
                  n3046 = property on="Engage" class="Bool (strict)"("Boolean Text.Text"=w4319) -> ()  [unwired: 2 in, 2 out]
                }
                frame 27 {
                  n3047 = property on="Boolean  4" class="Bool (strict)"("Boolean Text.Text"=w4320) -> ()  [unwired: 2 in, 2 out]
                }
                frame 28 {
                  n3048 = property on="Test \nStatus" class="Bool (strict)"("Boolean Text.Text"=w4321) -> ()  [unwired: 2 in, 2 out]
                }
                frame 29 {
                }
                frame 30 {
                }
                frame 31 {
                  n3049 = property on="FF Calibration g" class="WFGraph (strict)"("X Scale.Name Label.Text"=w4322) -> ()  [unwired: 2 in, 2 out]
                }
                frame 32 {
                  n3050 = property on="RSTCOF" class="Bool"("Boolean Text.Text"=w4323) -> ()  [unwired: 2 in, 2 out]
                  n3051 = property on="RST FF" class="Bool"("Boolean Text.Text"=w4323) -> ()  [unwired: 2 in, 2 out]
                  n3052 = property on="RST TEMP" class="Bool"("Boolean Text.Text"=w4323) -> ()  [unwired: 2 in, 2 out]
                  n3053 = property on="RSTV1 3" class="Bool"("Boolean Text.Text"=w4323) -> ()  [unwired: 2 in, 2 out]
                  n3054 = property on="rstv2" class="Bool"("Boolean Text.Text"=w4323) -> ()  [unwired: 2 in, 2 out]
                  n3055 = property on="RSTV1 2" class="Bool"("Boolean Text.Text"=w4323) -> ()  [unwired: 2 in, 2 out]
                  n3056 = property on="RST CP" class="Bool"("Boolean Text.Text"=w4323) -> ()  [unwired: 2 in, 2 out]
                }
                frame 33 {
                  "S 61" <- w4324
                }
                frame 34 {
                  "String 23" <- w4325
                }
                frame 35 {
                  n3057 = property on="Rh Before" class="DigNum (strict)"("Caption.Text"=w4326) -> ()  [unwired: 2 in, 2 out]
                }
                frame 36 {
                  n3058 = Match Pattern(string=w4327, regular expression=",") -> (before substring=→"bs":string, after substring=→"as":string)  [unwired: 1 in, 2 out]
                  n3059 = property on="Rh After" class="DigNum (strict)"("Caption.Text"=w4327) -> ()  [unwired: 2 in, 2 out]
                }
                frame 37 {
                  n3060 = Match Pattern(string=w4336, regular expression=",") -> (before substring=w4335:string, after substring=w4334:string)  [unwired: 1 in, 2 out]
                  "bs" <- w4335
                  "as" <- w4334
                  n3061 = Concatenate Strings(w4335, w4334) -> (w4331:string)
                  n3062 = property on="Humidity before test 2" class="DigNum (strict)"("Caption.Text"=w4331) -> ()  [unwired: 2 in, 2 out]
                  n3063 = property on="Humidity before test" class="DigNum (strict)"("Caption.Text"=w4331) -> ()  [unwired: 2 in, 2 out]
                  n3064 = Concatenate Strings(w4331, "=" ("string")) -> (w4332:string)
                  n3065 = local write "S 38"(w4332) -> ()
                }
                frame 38 {
                  n3066 = Match Pattern(string=w4343, regular expression=",") -> (before substring=w4342:string, after substring=w4341:string)  [unwired: 1 in, 2 out]
                  "bs" <- w4342
                  "as" <- w4341
                  n3067 = Concatenate Strings(w4342, w4341) -> (w4338:string)
                  n3068 = property on="Humidity after test 2" class="DigNum (strict)"("Caption.Text"=w4338) -> ()  [unwired: 2 in, 2 out]
                  n3069 = Concatenate Strings(w4338, "=" ("string")) -> (w4340:string)
                  n3070 = property on="Humidity after test" class="DigNum (strict)"("Caption.Text"=w4338) -> ()  [unwired: 2 in, 2 out]
                  n3071 = local write "S 39"(w4340) -> ()
                }
                frame 39 {
                  n3072 = Match Pattern(string=w4350, regular expression=",") -> (before substring=w4349:string, after substring=w4348:string)  [unwired: 1 in, 2 out]
                  "bs" <- w4349
                  "as" <- w4348
                  n3073 = Concatenate Strings(w4349, w4348) -> (w4345:string)
                  n3074 = property on="Temperature before test 2" class="DigNum (strict)"("Caption.Text"=w4345) -> ()  [unwired: 2 in, 2 out]
                  n3075 = property on="Temperature before test" class="DigNum (strict)"("Caption.Text"=w4345) -> ()  [unwired: 2 in, 2 out]
                  n3076 = Concatenate Strings(w4345, "=" ("string")) -> (→"String 34":string)
                }
                frame 40 {
                  n3077 = Match Pattern(string=w4357, regular expression=",") -> (before substring=w4356:string, after substring=w4355:string)  [unwired: 1 in, 2 out]
                  "bs" <- w4356
                  "as" <- w4355
                  n3078 = Concatenate Strings(w4356, w4355) -> (w4352:string)
                  n3079 = property on="Temperature after test 2" class="DigNum (strict)"("Caption.Text"=w4352) -> ()  [unwired: 2 in, 2 out]
                  n3080 = Concatenate Strings(w4352, "=" ("string")) -> (→"String 35":string)
                  n3081 = property on="Temperature after test" class="DigNum (strict)"("Caption.Text"=w4352) -> ()  [unwired: 2 in, 2 out]
                }
                frame 41 {
                  n3082 = property on="AVP" class="DigNum (strict)"("Caption.Text"=w4361) -> ()  [unwired: 2 in, 2 out]
                  n3083 = property on="AVP 2" class="DigNum (strict)"("Caption.Text"=w4361) -> ()  [unwired: 2 in, 2 out]
                  n3084 = Concatenate Strings(w4361, "=" ("string")) -> (→"String 36":string)
                }
                frame 42 {
                  n3085 = property on="MWSD" class="DigNum (strict)"("Caption.Text"=w4364) -> ()  [unwired: 2 in, 2 out]
                  n3086 = property on="MWSD 2" class="DigNum (strict)"("Caption.Text"=w4364) -> ()  [unwired: 2 in, 2 out]
                  n3087 = Concatenate Strings(w4364, "=" ("string")) -> (→"String 37":string)
                }
                frame 43 {
                  n3088 = property on="HCF 2" class="DigNum (strict)"("Caption.Text"=w4367) -> ()  [unwired: 2 in, 2 out]
                  n3089 = property on="HCF" class="DigNum (strict)"("Caption.Text"=w4367) -> ()  [unwired: 2 in, 2 out]
                  n3090 = Concatenate Strings(w4367, "=" ("string")) -> (→"String 38":string)
                }
                frame 44 {
                  n3091 = Concatenate Strings(w4369, "=" ("string")) -> (→"String 39":string)
                  n3092 = property on="WS1.4 2" class="DigNum (strict)"("Caption.Text"=w4369) -> ()  [unwired: 2 in, 2 out]
                  n3093 = property on="WS1.4" class="DigNum (strict)"("Caption.Text"=w4369) -> ()  [unwired: 2 in, 2 out]
                }
                frame 45 {
                  n3094 = property on="Save Results" class="Bool (strict)"("Boolean Text.Text"=w4371) -> ()  [unwired: 2 in, 2 out]
                }
                frame 46 {
                  n3095 = local write "S 47"(w4372) -> ()
                }
                frame 47 {
                  n3096 = local write "S 48"(w4373) -> ()
                }
                frame 48 {
                  n3097 = local write "S 49"(w4374) -> ()
                }
                frame 49 {
                  n3098 = local write "S 50"(w4375) -> ()
                }
                frame 50 {
                  n3099 = local write "S 51"(w4376) -> ()
                }
                frame 51 {
                  n3100 = local write "S 52"(w4377) -> ()
                }
                frame 52 {
                  n3101 = local write "S 53"(w4378) -> ()
                }
                frame 53 {
                  n3102 = local write "S 54"(w4379) -> ()
                }
                frame 54 {
                  n3103 = local write "S 55"(w4380) -> ()
                }
                frame 55 {
                  n3104 = local write "S 56"(w4381) -> ()
                }
                frame 56 {
                  n3105 = local write "S 57"(w4382) -> ()
                }
                frame 57 {
                  n3106 = local write "S 58"(w4383) -> ()
                }
                frame 58 {
                  n3107 = local write "S 59"(w4384) -> ()
                }
                frame 59 {
                  n3108 = local write "S 60"(w4385) -> ()
                }
                frame 60 {
                  n3109 = local write "S 62"(w4386) -> ()
                }
                frame 61 {
                  n3110 = local write "S 63"(w4387) -> ()
                }
                frame 62 {
                  n3111 = local write "S 64"(w4388) -> ()
                }
                frame 63 {
                  n3112 = local write "S 65"(w4389) -> ()
                }
                frame 64 {
                  n3113 = local write "S 66"(w4390) -> ()
                }
                frame 65 {
                  n3114 = local write "S 67"(w4391) -> ()
                }
                frame 66 {
                  n3115 = local write "S 68"(w4392) -> ()
                }
                frame 67 {
                  n3116 = local write "S 69"(w4393) -> ()
                }
                frame 68 {
                  n3117 = local write "S 70"(w4394) -> ()
                }
                frame 69 {
                  n3118 = local write "S 71"(w4395) -> ()
                }
                frame 70 {
                  n3119 = local write "S 72"(w4396) -> ()
                }
                frame 71 {
                  n3120 = local write "S 73"(w4397) -> ()
                }
                frame 72 {
                  n3121 = local write "S 74"(w4398) -> ()
                }
                frame 73 {
                  n3122 = local write "S 75"(w4399) -> ()
                }
                frame 74 {
                  n3123 = local write "S 76"(w4400) -> ()
                }
                frame 75 {
                  n3124 = local write "S 77"(w4401) -> ()
                }
                frame 76 {
                  n3125 = local write "S 78"(w4402) -> ()
                }
                frame 77 {
                  n3126 = local write "S 79"(w4403) -> ()
                }
                frame 79 {
                  n3127 = property on="Sample Temperature ( °C )" class="XYGraph (strict)"("Y Scale.Name Label.Text"=w4404) -> ()  [unwired: 2 in, 2 out]
                }
                frame 80 {
                  n3128 = local write "S 81"(w4405) -> ()
                  n3129 = property on="Humidity ( %Rh )" class="XYGraph (strict)"("Y Scale.Name Label.Text"=w4405) -> ()  [unwired: 2 in, 2 out]
                }
                frame 78 {
                  n3130 = property on="Air Temperature  ( °C )" class="XYGraph (strict)"("X Scale.Name Label.Text"=w4406) -> ()  [unwired: 2 in, 2 out]
                  n3131 = property on="Humidity ( %Rh )" class="XYGraph (strict)"("X Scale.Name Label.Text"=w4406) -> ()  [unwired: 2 in, 2 out]
